vi "mainVI_1.vi"() -> ()   [LabVIEW 2019]
panel:
  out "Waveform Graph":dbl[][](graph)
  in  "New plot":bool
  in  "stop":bool
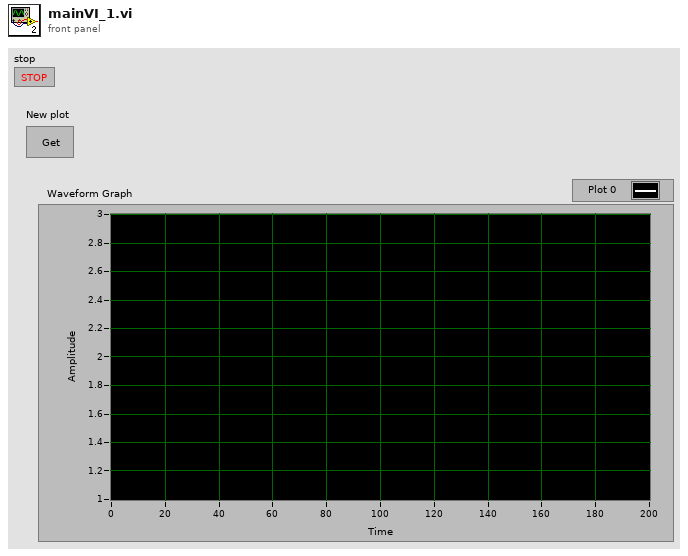
[diagram p1: front panel]
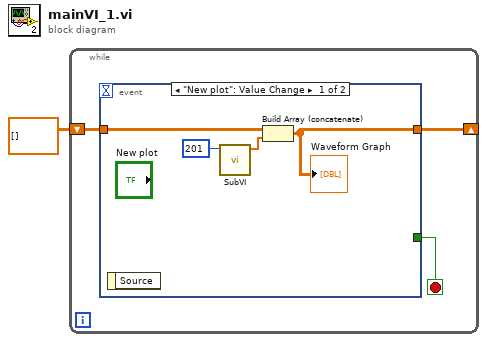
[diagram p0: block diagram]
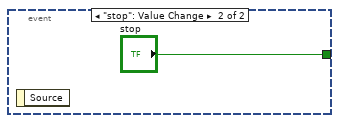
[diagram p2: hidden frame]
diagram:
  n1 = while {
    shift-right: [w4] -> _
    shift-left: dbl[][] [] -> [w3]
    stop <- w2 stop-if-true
    n2 = event shown="[0] \"New plot\": Value Change" {
      selector: _ -> [_ _]
      dyn-events: _ -> [_ _]
      timeout: _ -> [_ _]
      tunnel: [w6 _] -> w4
      tunnel: w3 -> [w5 _]
      tunnel: [_ "stop"] -> w2
      event "New plot": Value Change {
        n3 = event-data() -> ()  [unwired: 1 in, 1 out]
        n4 = call "SubVI.vi"("Points"=201) -> ("Disorder Pattern 2"=w7:dbl[])  [unwired: 10 in]
        n5 = Build Array (concatenate)(w5, w7) -> (w6:dbl[][])
        "Waveform Graph" <- w6
      }
      event "stop": Value Change {
        n6 = event-data() -> ()  [unwired: 1 in, 1 out]
      }
    }
  }
